vi "Save config.vi"(8 "error in (no error)":errorcluster, 10 "Temperature":dbl, 11 "DAQ Device Name":tag) -> (0 "error out":errorcluster)   [LabVIEW 2020, in "UI.lvlib"]
uses:
  UI.lvlib
  <vilib>/Utility/file.llb/Application Directory.vi
  <vilib>/Utility/config.llb/Write Key (String).vi
  <vilib>/Utility/config.llb/Write Key (Double).vi
  <vilib>/Utility/config.llb/NI_LVConfig.lvlib
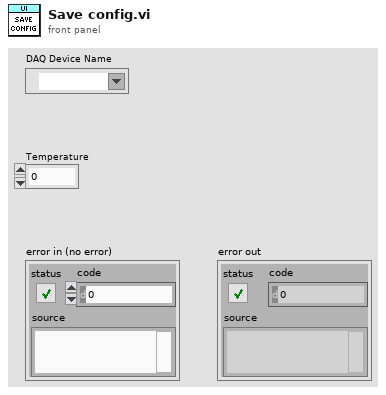
[diagram p1: front panel]
types:
  T1 = typedef "NI_LVConfig.lvlib/Config Data RefNum.ctl" = refnum<k1>
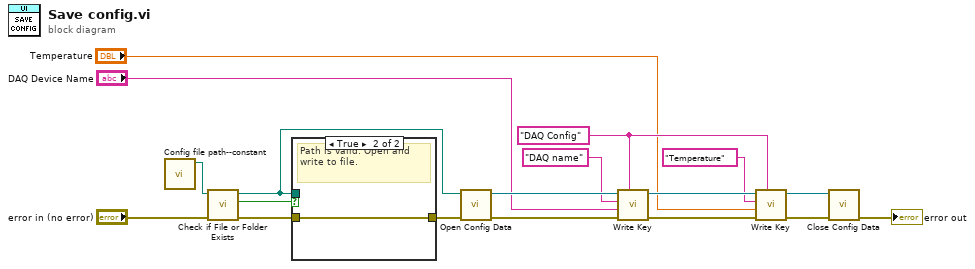
[diagram p0: block diagram]
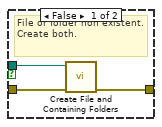
[diagram p2: hidden frame]
diagram:
  w3 = "DAQ Config" ("section")
  n1 = call "Config file path--constant.vi"() -> ("Path"=w16:path)  [unwired: 11 in]
  n2 = call <vilib>:"Check if File or Folder Exists.vi"("error in (no error)"="error in (no error)", "path"=w16) -> ("error out"=w13:errorcluster, "file or folder exists?"=w12:bool, "dup path"=w10:path)  [unwired: 7 in]
  n3 = case shown="True" w12 {
    tunnel: w13 -> [w21 w22]
    tunnel: w10 -> [w19 _]
    tunnel: [w20 w22] -> w11
    frame False {
      # "File or folder non existent. Create both."
      n4 = call <vilib>:"Create File and Containing Folders.vi"("error in (no error)"=w21, "file path"=w19) -> ("error out"=w20:errorcluster)  [unwired: 8 in, 1 out]
    }
    frame True {
      # "Path is valid. Open and write to file."
    }
  }
  n5 = call <vilib>:"Open Config Data.vi"("error in (no error)"=w11, "configuration file path"=w10) -> ("error out"=w9:errorcluster, "refnum"=w15:T1)  [unwired: 7 in, 1 out]
  n6 = call-poly <vilib>:"Write Key.vi"("section"=w3, "error in (no error)"=w9, "value"="DAQ Device Name", "key"="DAQ name", "refnum"=w15) -> ("error out"=w7:errorcluster, "refnum out"=w5:T1)  [unwired: 4 in, 1 out]
  n7 = call-poly <vilib>:"Write Key.vi"("section"=w3, "error in (no error)"=w7, "value"="Temperature", "key"="Temperature", "refnum"=w5) -> ("error out"=w6:errorcluster, "refnum out"=w4:T1)  [unwired: 4 in, 1 out]
  n8 = call <vilib>:"Close Config Data.vi"("error in (no error)"=w6, "refnum"=w4) -> ("error out"=→"error out":errorcluster)  [unwired: 8 in, 1 out]
